vi "Periodic Tasks.vi"(8 "error in":errorcluster) -> ()   [LabVIEW 2016]
doc: "This VI runs in parallel to other tasks. It can contain as many user-defined periodic loops as you need. These can carry out PID or other sorts of timed response."
uses:
  <vilib>/addons/control/pid/pid.llb/PID Structure.ctl
  <vilib>/addons/control/pid/pid.llb/PID Time Unit.ctl
  <vilib>/addons/control/pid/pid.llb/PID Gain Unit.ctl
  Control 1.ctl
  <vilib>/Rock Robotics/WPI/ThirdParty/CanMotor/TalonSRX/WPI_CANTalonSRX_StatusFrame.ctl
  <vilib>/Rock Robotics/WPI/Solenoid/WPI_SolenoidValue.ctl
  <vilib>/Rock Robotics/WPI/Utilities/WPI_GetSetVariantRefNum.vi
  <vilib>/addons/control/pid/pid.llb/PID Structure Conversion (DBL).vi
  Robot Global Data.vi
  <vilib>/addons/control/pid/pid.llb/PID (DBL).vi
  <vilib>/addons/control/pid/pid.llb/PID Output Rate Limiter (DBL).vi
  <vilib>/Rock Robotics/WPI/RobotDrive/WPI_RobotDriveArcadeDrive_Standard(NoSaturation).vi
  <vilib>/Rock Robotics/Network Tables/NT Write Numeric Array.vi
  <vilib>/Rock Robotics/Network Tables/NT Write Number.vi
  <vilib>/Rock Robotics/Network Tables/NT Write Boolean.vi
  <vilib>/Rock Robotics/WPI/Solenoid/WPI_SolenoidSetEnum.vi
  <vilib>/Rock Robotics/WPI/Solenoid/Deprecated/WPI_SolenoidGetBool.vi
  <vilib>/addons/control/pid/NI_PID_pid.lvlib
panel:
  in  "BallIntakeCmd":dbl=0.45
  out "ANG-Input":dbl format="%#_3g"
  out "ANG-Output":dbl format="%#_3g"
  out "FWD-Output":dbl format="%#_3g"
  out "FWD-Input":dbl format="%#_3g"
  in  "ANG-A":dbl(slide)=0.7572815533980581 scale=0.0..1.0
  in  "ANG-B":dbl(slide)=0.3058252427184466 scale=0.0..1.0
  in  "FWD-B":dbl(slide)=0.24757281553398056 scale=0.0..1.0
  in  "FWD-A":dbl(slide)=0.12135922330097086 scale=0.0..1.0
  in  "DT Encoder Reset":bool
  in  "GearIntakeCmd":dbl=0.8
  in  "ShooterFlywCmd":dbl=8320.0
  in  "CtrlConv+UptReverse":bool
  in  "CtrlIntakeReverse":bool
  out "Flywheel Cmd & Speed":cluster{"Sensor Velocity":dbl}(graph)
  out "DTLeft - Under Voltage":bool
  out "DTLeft - Over Temp 2":bool
  out "DTRight- Over Temp":bool
  out "DTRight- Under Voltage":bool
  in  "output rate (EGU/min)":dbl=10000.0 format="%.2f"
  in  "P Fly":dbl=0.4
  in  "I Fly":dbl
  in  "D Fly":dbl
  in  "F Fly":dbl
  out "ShooterFlywThrottle":dbl
  out "ShooterFlywCur":dbl
  out "ShooterFlywEncVel":dbl
  out "ShooterFlywEncPos":dbl
  out "ShooterMasSensorVel":dbl
  out "ShooterFlywError":dbl
  in  "ShooterUptakeCmd":dbl=0.5
  out "ShooterUptakeSelection":bool
  out "ShooterUpCurr":dbl
  out "ShooterUpThrottle":dbl
  in  "ConveyorCmd":dbl=0.95
  out "DT Right Distance":dbl
  out "DT Encoder Avg":dbl
  out "Yaw Cmd & Angle":cluster{"Drive Angle":dbl, "Yaw":dbl}(graph)={"Drive Angle"=0.0, "Yaw"=-0.012991420041388195}
  out "PID gains F":T1
  out "PID gains A":T1
  out "DT Left/Right Motors":T2(graph)
  out "Arcade Y-Axis":dbl
  out "Arcade X-Axis":dbl
  out "Angle PID Out":dbl(graph)
  out "Fwd PID Out":dbl(graph)
  in  "Y-AxisJoyWgt":dbl=1.0
  in  "Fwd PID On":bool
  out "Fwd PIDoutput":dbl
  in  "PIDoutputRange F":cluster{"output high":dbl, "output low":dbl}={"output high"=0.8, "output low"=-0.8} {"output low" format="%.2f"; "output high" format="%.2f"}
  in  "ResetPID F":bool
  in  "derivative unit F":T3 items=["min", "s"]
  in  "proportional unit F":T4 items=["Gain (K)", "Band (PB)"]
  in  "integral unit F":T3 items=["min", "s"]
  in  "derivative F":dbl=4e-06
  in  "integral F":dbl=0.2
  in  "proportional F":dbl=0.002
  in  "Fwd PID structure":T5=1 items=["Academic (Standard)", "Parallel", "Series"]
  out "Angle PIDoutput":dbl
  in  "PIDoutputRange A":cluster{"output high":dbl, "output low":dbl}={"output high"=0.7, "output low"=-0.7} {"output low" format="%.2f"; "output high" format="%.2f"}
  in  "ResetAngle PID":bool
  in  "derivative unit A":T3 items=["min", "s"]
  in  "proportional unit A":T4 items=["Gain (K)", "Band (PB)"]
  in  "integral unit A":T3 items=["min", "s"]
  in  "derivative A":dbl=5e-05
  in  "integral A":dbl=11.0
  in  "proportional A":dbl=0.05
  in  "Angle PID structure":T5=1 items=["Academic (Standard)", "Parallel", "Series"]
  in  "DriveDistance Cmd":dbl
  out "DT Fwd Cmd & Right Encoder":cluster{"Drive Angle":dbl, "Yaw":dbl}(graph)={"Drive Angle"=0.0, "Yaw"=-0.012991420041388195}
  in  "Reset Gyro":bool
  out "Gyro Angle":dbl
  out "DT Left Distance":dbl
  out "DT Fwd Cmd & Left Encoder":cluster{"Drive Angle":dbl, "Yaw":dbl}(graph)={"Drive Angle"=0.0, "Yaw"=-0.012991420041388195}
  out "DT Encoder L-R":dbl(graph)
  out "DT Forward Cmd & Avg Distance":cluster{"Drive Angle":dbl, "Yaw":dbl}(graph)={"Drive Angle"=0.0, "Yaw"=-0.012991420041388195}
  out "Motor Values":dbl[](array[numeric])
  in  "X-AxisJoyWgt":dbl=0.8
  in  "Angle PID On":bool
  out "DTGearShiftHi":bool
  in  "DTClearStickyFaults":bool
  in  "DriveAngleCmd":dbl
  # "JOYSTICK SENSITIVITY COMPENSATION"
  # "P=0.025"
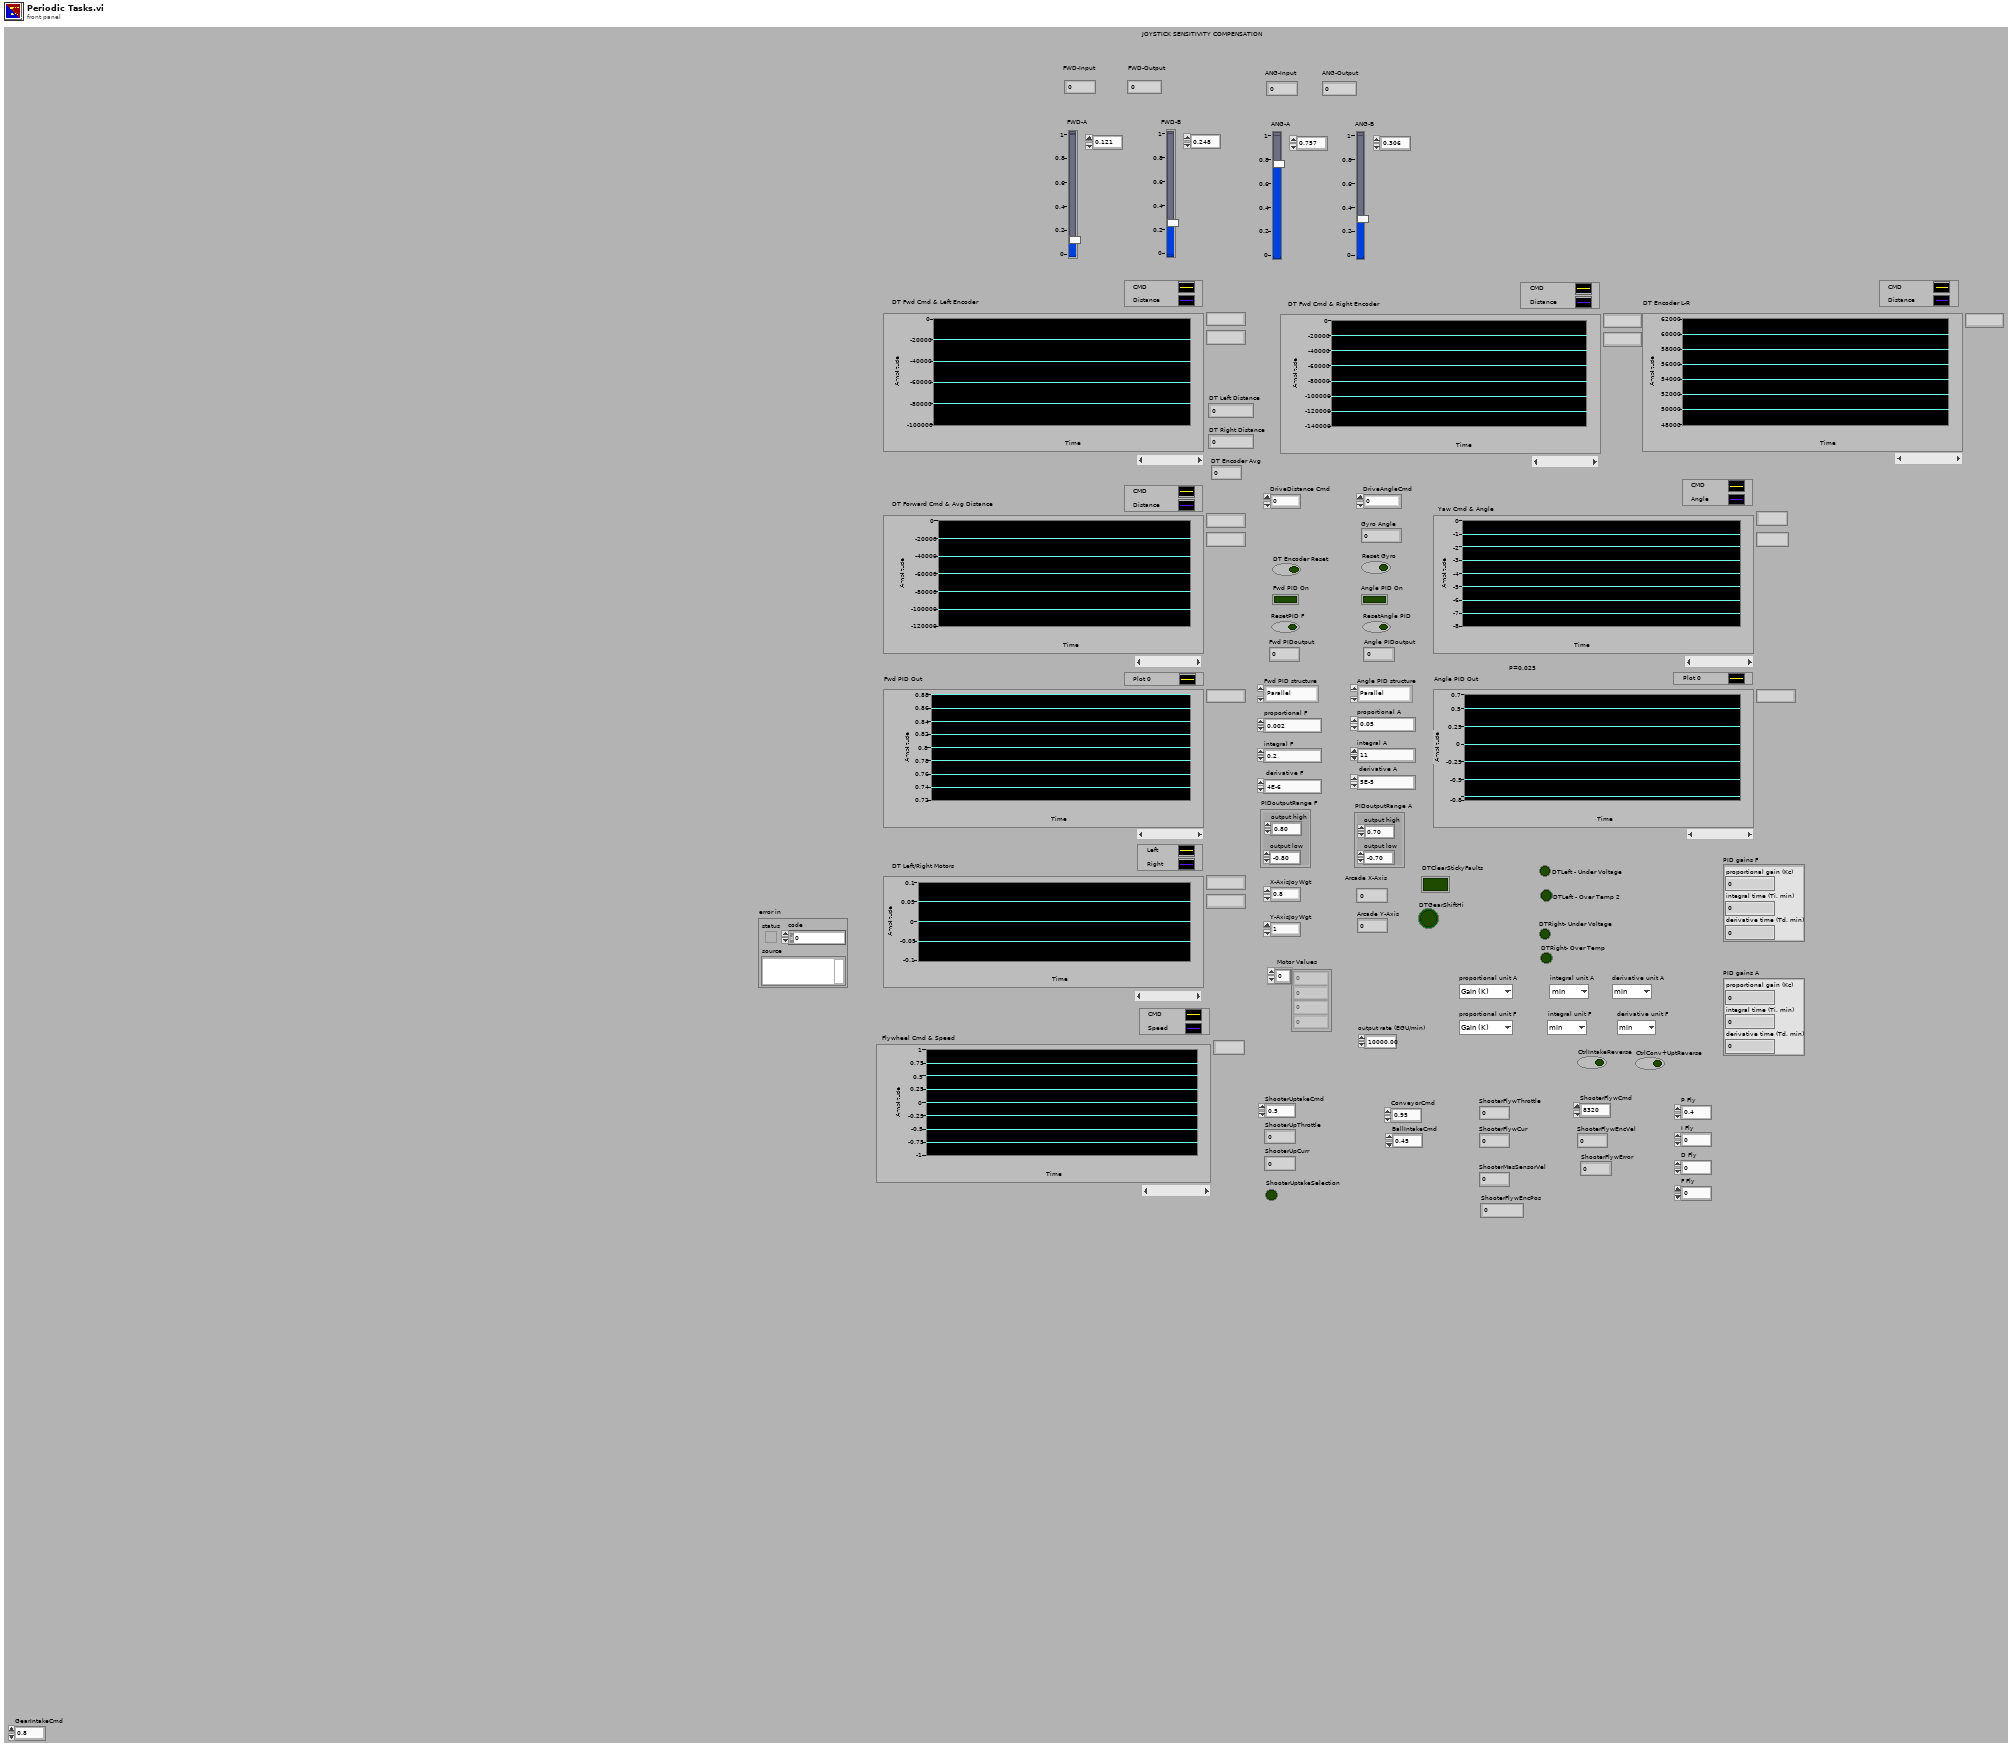
[diagram p1: front panel]
types:
  T1 = cluster{"proportional gain (Kc)":dbl, "integral time (Ti, min)":dbl, "derivative time (Td, min)":dbl}
  T2 = cluster{"Motor Values[0]":dbl, "Motor Values[1]":dbl}
  T3 = typedef "NI_PID_pid.lvlib/PID Time Unit.ctl" = u16
  T4 = typedef "NI_PID_pid.lvlib/PID Gain Unit.ctl" = u16
  T5 = typedef "NI_PID_pid.lvlib/PID Structure.ctl" = u16
  T6 = typedef "WPI_MotorControlDeviceRef.ctl" = cluster{"DeviceStatus":errorcluster, "Type":T7, "PWM":cluster{"PWM Channel":T8, "DeadBand":T9}, "CAN":cluster{"Device Number":u8, "SetOutput VI Ref":variant, "GetOutput VI Ref":variant, "Enable VI Ref":variant, "Disable VI Ref":variant, "Data":variant}, "Invert":bool}
  T7 = typedef "WPI_MotorControlType.ctl" = enum16{"PWM", "CAN"}
  T8 = typedef "FPGA_DIOPWMChannel.ctl" = enum8{"PWM 0", "PWM 1", "PWM 2", "PWM 3", "PWM 4", "PWM 5", "PWM 6", "PWM 7", "PWM 8", "PWM 9", "PWM MXP 0", "PWM MXP 1", "PWM MXP 2", "PWM MXP 3", "PWM MXP 4", "PWM MXP 5", "PWM MXP 6", "PWM MXP 7", "PWM MXP 8", "PWM MXP 9", "Invalid"}
  T9 = typedef "WPI_PWMDeadband.ctl" = cluster{"Name":string, "maxPositivePwm":i32, "minPositivePwm":i32, "centerPwm":i32, "maxNegativePwm":i32, "minNegativePwm":i32, "angularRange":u16}
  T10 = typedef "WPI_JoystickDevRef.ctl" = cluster{"Device":T11}
  T11 = typedef "WPI_JoystickDeviceEnum.ctl" = enum16{"USB 0", "USB 1", "USB 2", "USB 3", "USB 4", "USB 5"}
  T12 = typedef "WPI_RobotDriveDevRef.ctl" = cluster{"DevStatus":errorcluster, "Motors[]":T6[], "Square Inputs":bool, "Max Output":dbl}
  T13 = cluster{"MotorControlDevRef":T6, "JoystickDevRef":T10, "RobotDriveDevRef":T12}
  T14 = typedef "WPI_SolenoidDevRef.ctl" = cluster{"DevStatus":errorcluster, "Pneumatics Control Module":u8, "Forward Solenoid Channel":T15, "Reverse Solenoid Channel":T15}
  T15 = typedef "WPI_SolenoidChannel.ctl" = enum8{"Solenoid 0", "Solenoid 1", "Solenoid 2", "Solenoid 3", "Solenoid 4", "Solenoid 5", "Solenoid 6", "Solenoid 7", "Invalid"}
  T16 = typedef "WPI_GyroDevRef.ctl" = cluster{"DevStatus":errorcluster, "Analog Channel":T17, "Offset":dbl, "Gain (VoltsPerDegree/Second)":dbl, "Gyro Type":enum16{"Analog", "XRS450"}, "Handle":i32, "SPI Bus":T18, "Device Found":bool, "Sample Rate":dbl, "Calibrate On Open":bool}
  T17 = typedef "FPGA_AIChannel.ctl" = enum8{"AI 0", "AI 1", "AI 2", "AI 3", "AI MXP 0", "AI MXP 1", "AI MXP 2", "AI MXP 3", "Invalid"}
  T18 = typedef "spi_bus.ctl" = enum16{"SPI On-Board, CS0", "SPI On-Board, CS1", "SPI On-Board, CS2", "SPI On-Board, CS3", "SPI MXP", "Invalid"}
  T19 = typedef "WPI_SolenoidValue.ctl" = enum16{"Off", "On", "Forward", "Reverse"}
  T20 = typedef "WPI_CANTalonSRX_GlobalStatus.ctl" = cluster{"Applied Throttle":dbl, "Module Enabled":bool, "CAN Error":errorcluster, "Closed Loop Error":dbl, "Forward Limit Switch Closed":bool, "Reverse Limit Switch Closed":bool, "Sensor Position":dbl, "Sensor Velocity":dbl, "Current":dbl, "Sticky Fault - Over Temp":bool, "Sticky Fault - Under Voltage":bool, "Sticky Fault - Forward Limit":bool, "Sticky Fault - Reverse Limit":bool, "Sticky Fault - Forward Soft Limit":bool, "Sticky Fault - Reverse Soft Limit":bool, "Brake is Enabled":bool, "Encoder Position":dbl, "Encoder Velocity":dbl, "Encoder Index Count":dbl, "Encoder A Pin State":bool, "Encoder B Pin State":bool, "Encoder Index Pin State":bool, "Analog In":dbl, "Analog In Velocity":dbl, "Temperature (C)":dbl, "Battery Voltage":dbl, "Control 5 Is Supported":bool, "Current Profile Slot Select":dbl, "Pos Div 8":bool, "Vel Div 4":bool, "Pulse Width Position":i32, "Pulse Width Velocity":i32, "Pulse Width Rise To Rise (us)":i32, "Pulse Width Rise To Fall (us)":i32, "Mot Prof Active Is Under Run":bool, "Mot Prof Active Has Under Run":bool, "Mot Prof Active Is Last":bool, "Mot Prof Active Velocity Only":bool, "Mot Prof Active Is Valid":bool, "Mot Prof Buffer Is Full":bool, "Mot Prof Active Profile Slot Select":i32, "Mot Prof NextID":i32, "Mot Prof Count":i32, "Mot Prof Active Velocity":dbl, "Mot Prof Active Position":dbl, "Mot Prof Output Enable":i32}
  T21 = cluster{"Motor Values[0]":dbl, "Motor Values[1]":dbl, "Motor Values[2]":dbl, "Motor Values[3]":dbl, "Motor Values[4]":dbl, "Motor Values[5]":dbl, "Motor Values[6]":dbl, "Motor Values[7]":dbl, "Motor Values[8]":dbl}
  T22 = enum16{"Start", "Search", "Secure", "Release", "Standby", "Wait", "Wait Release"}
  T23 = typedef "Control 1.ctl" = enum16{"Autonomous Disabled", "Autonomous Enabled", "Teleop Disabled", "Teleop Enabled", "Disconnected", "Finish", "Test Disabled", "Test Enabled", "Emergency Stopped"}
  T24 = cluster{"Buttons[0]":bool, "Buttons[1]":bool, "Buttons[2]":bool, "Buttons[3]":bool, "Buttons[4]":bool, "Buttons[5]":bool, "Buttons[6]":bool, "Buttons[7]":bool, "Buttons[8]":bool}
  T25 = cluster{"Axes[0]":dbl, "Axes[1]":dbl, "Axes[2]":dbl, "Axes[3]":dbl, "Axes[4]":dbl, "Axes[5]":dbl, "Axes[6]":dbl, "Axes[7]":dbl, "Axes[8]":dbl}
  T26 = typedef "WPI_DriverStationRobotMode2.ctl" = enum16{"Autonomous Disabled", "Autonomous Enabled", "Teleop Disabled", "Teleop Enabled", "Disconnected", "Finish", "Test Disabled", "Test Enabled", "Emergency Stopped"}
  T27 = typedef "WPI_CANTalonSRX_StatusFrame.ctl" = enum16{"General Status Frame", "Feedback Status Frame", "Quadrature Status Frame", "Analog Temp Vbat Status Frame", "Pulse Width Status Frame"}
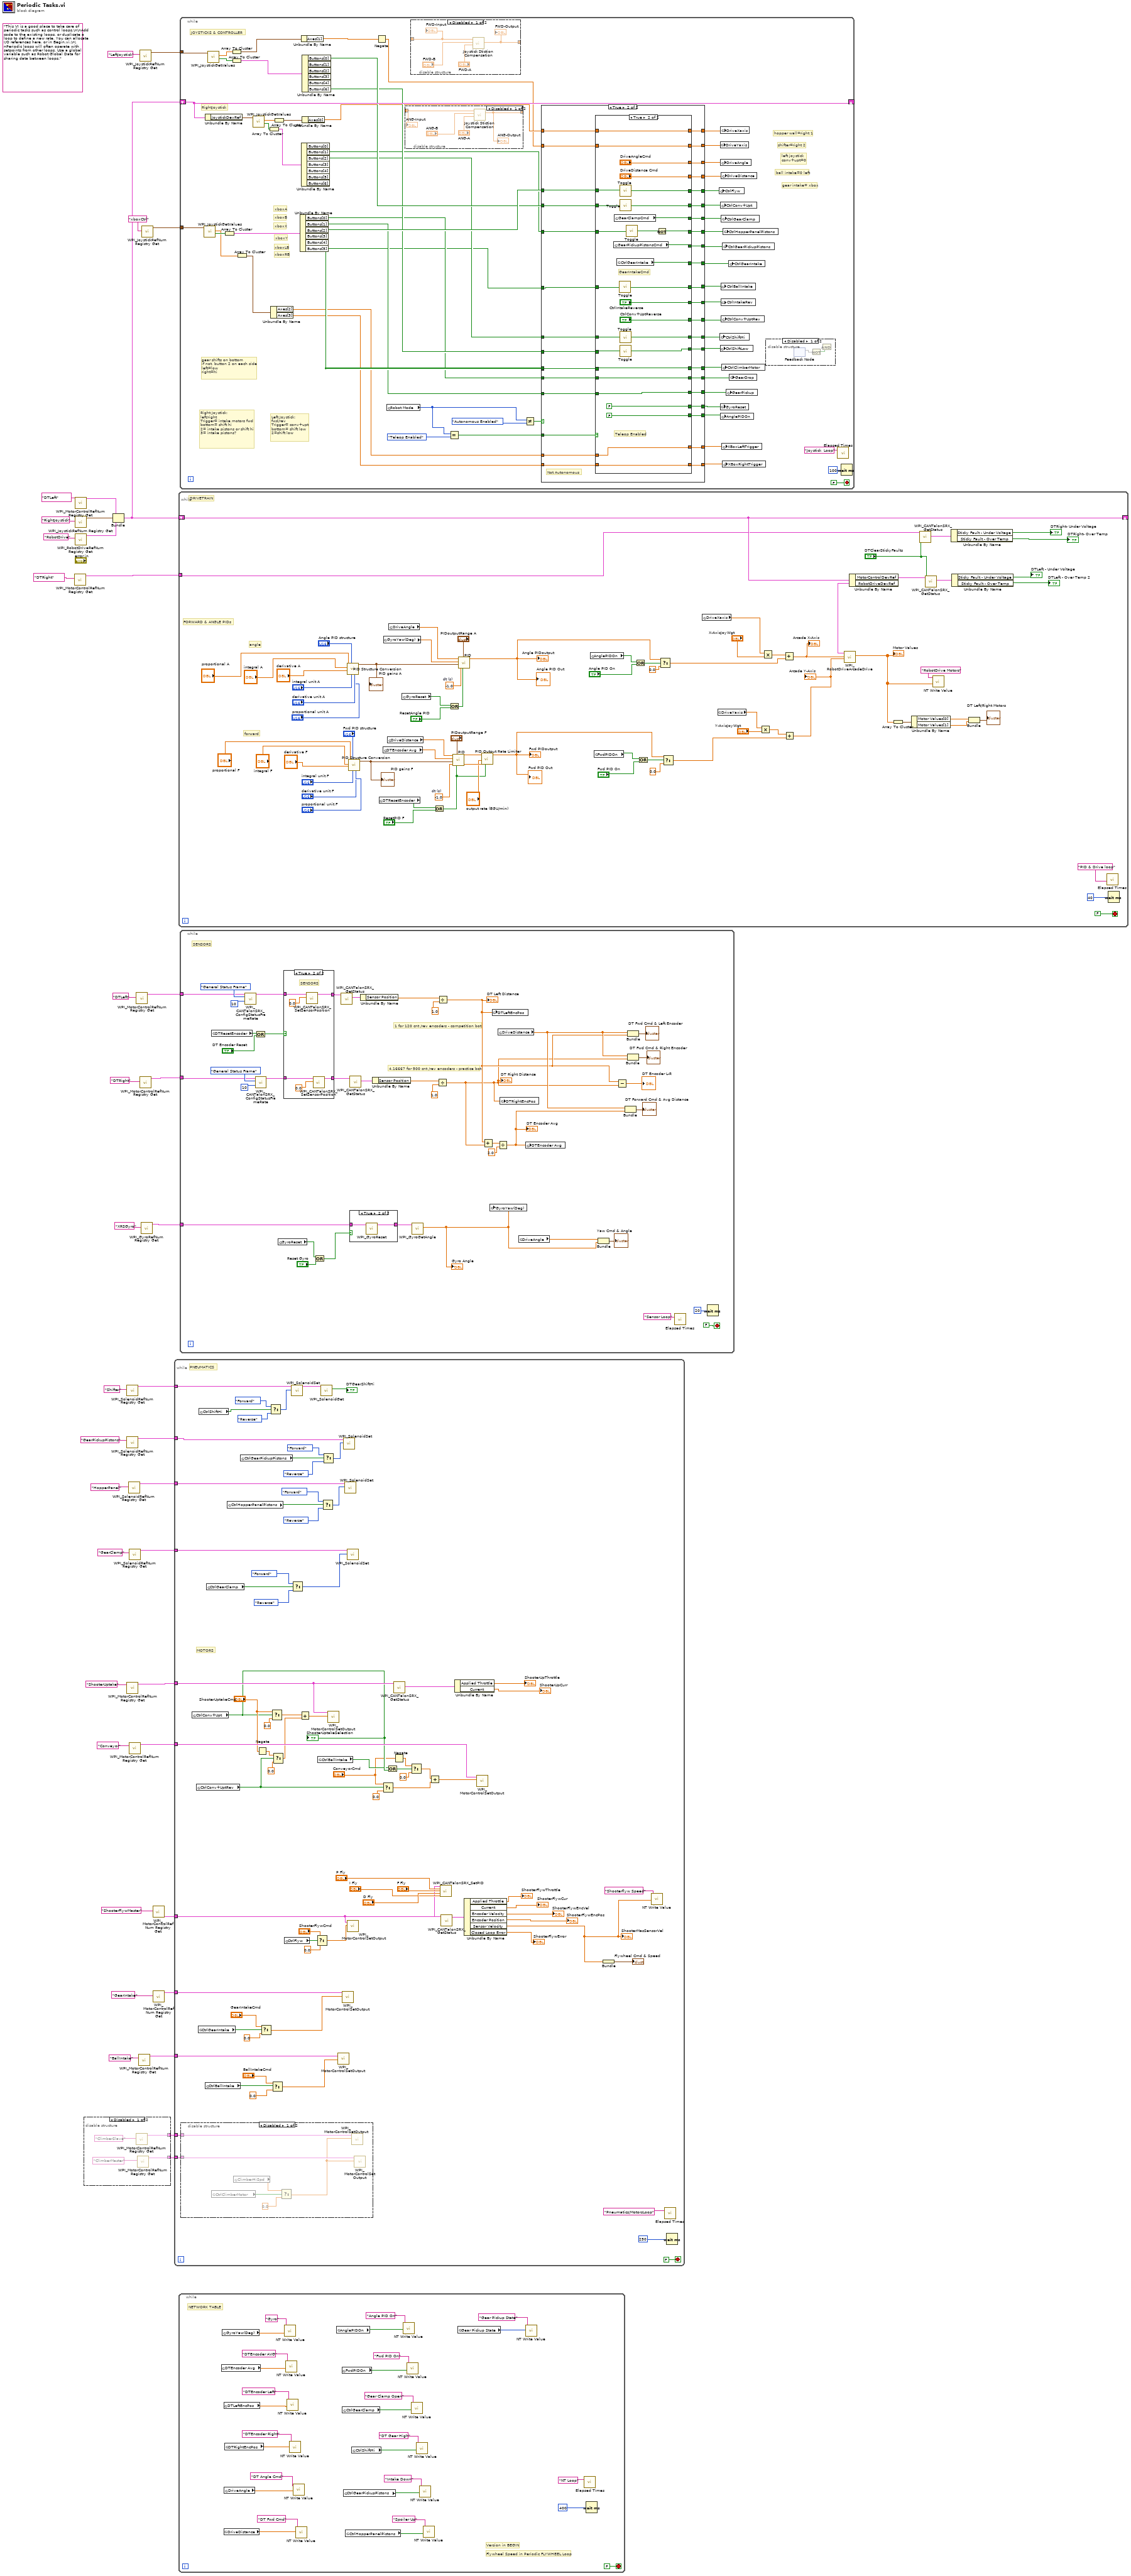
[diagram p0: block diagram]
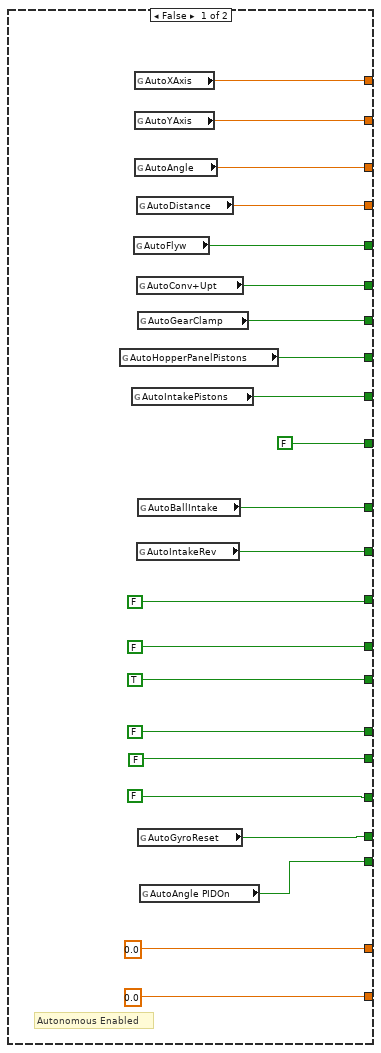
[diagram p9: hidden frame]
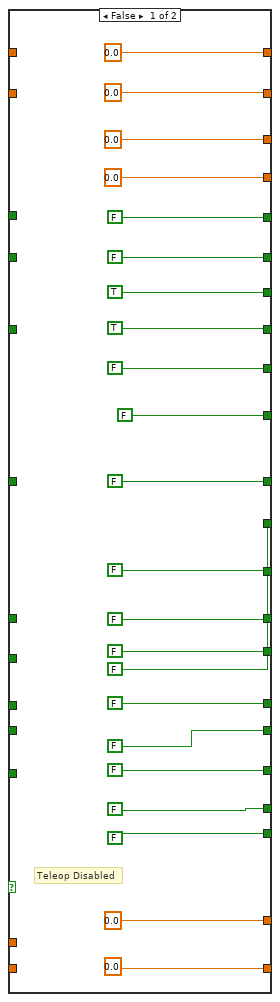
[diagram p10: hidden frame]
diagram:
  (unwired) "This VI is a good place to take care of periodic tasks such as control loops.\n\nAdd code to the existing loops, or duplicate a loop to define a new rate. You can allocate I/O references here, or in Begin.vi.\n\nPeriodic loops will often operate with setpoints from other loops. Use a global variable such as Robot Global Data for sharing data between loops."
  n1 = call <vilib>:"WPI_MotorControlRefNum Registry Get.vi"("refnum name"="DTRight") -> ("MotorControlDevRef"=w28:T6)  [unwired: 9 in, 1 out]
  n2 = call <vilib>:"WPI_MotorControlRefNum Registry Get.vi"("refnum name"="DTLeft") -> ("MotorControlDevRef"=w30:T6)  [unwired: 9 in, 1 out]
  n3 = call <vilib>:"WPI_JoystickRefNum Registry Get.vi"("refnum name"="RightJoystick") -> ("JoystickDevRef"=w37:T10)  [unwired: 1 in, 9 out]
  n4 = call <vilib>:"WPI_RobotDriveRefNum Registry Get.vi"("refnum name"="RobotDrive") -> ("RobotDriveDevRef"=w36:T12)  [unwired: 1 in, 9 out]
  n5 = disable-structure shown="Disabled" {
    disable-tunnel: [w41 _] -> w4
    disable-tunnel: [w40 _] -> w3
    frame Disabled {
      n6 = call <vilib>:"WPI_MotorControlRefNum Registry Get.vi"("refnum name"="ClimberSlave") -> ("MotorControlDevRef"=w41:T6)  [unwired: 9 in, 1 out]
      n7 = call <vilib>:"WPI_MotorControlRefNum Registry Get.vi"("refnum name"="ClimberMaster") -> ("MotorControlDevRef"=w40:T6)  [unwired: 9 in, 1 out]
    }
    frame Enabled {
    }
  }
  n8 = Bundle("MotorControlDevRef"=w30, "JoystickDevRef"=w37, "RobotDriveDevRef"=w36) -> (w35:T13)  [unwired: 1 out]
  n9 = call <vilib>:"WPI_SolenoidRefNum Registry Get.vi"("refnum name"="Shifter") -> ("SolenoidDevRef"=w25:T14)  [unwired: 9 in, 1 out]
  n10 = call <vilib>:"WPI_SolenoidRefNum Registry Get.vi"("refnum name"="GearPickupPistons") -> ("SolenoidDevRef"=w17:T14)  [unwired: 9 in, 1 out]
  n11 = call <vilib>:"WPI_MotorControlRefNum Registry Get.vi"("refnum name"="ShooterUptake") -> ("MotorControlDevRef"=w20:T6)  [unwired: 9 in, 1 out]
  n12 = call <vilib>:"WPI_SolenoidRefNum Registry Get.vi"("refnum name"="HopperPanel") -> ("SolenoidDevRef"=w23:T14)  [unwired: 9 in, 1 out]
  n13 = call <vilib>:"WPI_SolenoidRefNum Registry Get.vi"("refnum name"="GearClamp") -> ("SolenoidDevRef"=w15:T14)  [unwired: 9 in, 1 out]
  n14 = call <vilib>:"WPI_MotorControlRefNum Registry Get.vi"("refnum name"="Conveyor") -> ("MotorControlDevRef"=w19:T6)  [unwired: 9 in, 1 out]
  n15 = call <vilib>:"WPI_MotorControlRefNum Registry Get.vi"("refnum name"="DTLeft") -> ("MotorControlDevRef"=w9:T6)  [unwired: 9 in, 1 out]
  n16 = call <vilib>:"WPI_MotorControlRefNum Registry Get.vi"("refnum name"="BallIntake") -> ("MotorControlDevRef"=w1:T6)  [unwired: 9 in, 1 out]
  n17 = call <vilib>:"WPI_JoystickRefNum Registry Get.vi"("refnum name"="LeftJoystick") -> ("JoystickDevRef"=w33:T10)  [unwired: 1 in, 9 out]
  n18 = call <vilib>:"WPI_MotorControlRefNum Registry Get.vi"("refnum name"="DTRight") -> ("MotorControlDevRef"=w8:T6)  [unwired: 9 in, 1 out]
  n19 = call <vilib>:"WPI_GyroRefNum Registry Get.vi"("refnum name"="XRSGyro") -> ("GyroDevRef"=w11:T16)  [unwired: 9 in, 1 out]
  n20 = call <vilib>:"WPI_JoystickRefNum Registry Get.vi"("refnum name"="xboxCtrl") -> ("JoystickDevRef"=w26:T10)  [unwired: 1 in, 9 out]
  n21 = call <vilib>:"WPI_MotorControlRefNum Registry Get.vi"("refnum name"="ShooterFlywMaster") -> ("MotorControlDevRef"=w13:T6)  [unwired: 9 in, 1 out]
  n22 = call <vilib>:"WPI_MotorControlRefNum Registry Get.vi"("refnum name"="GearIntake") -> ("MotorControlDevRef"=w5:T6)  [unwired: 9 in, 1 out]
  n23 = while {
    tunnel: w25 -> [w122]
    tunnel: w23 -> [w121]
    tunnel: w20 -> [w120]
    tunnel: w19 -> [w119]
    tunnel: w17 -> [w118]
    tunnel: w15 -> [w117]
    tunnel: w13 -> [w116]
    tunnel: w5 -> [w115]
    tunnel: w4 -> [w114]
    tunnel: w3 -> [w113]
    tunnel: w1 -> [w112]
    stop <- FALSE stop-if-true
    # "PNEUMATICS"
    # "MOTORS"
    n24 = disable-structure shown="Disabled" {
      disable-tunnel: w114 -> [w128 _]
      disable-tunnel: w113 -> [w127 _]
      frame Disabled {
        n25 = global read "Robot Global Data.vi" "CtrlClimberMotor"() -> (w124:bool)
        n26 = global read "Robot Global Data.vi" "ClimberHiSpd"() -> (w125:dbl)
        n27 = Select(t=w125, s=w124, f=0.0) -> (s? t:f=w123:dbl)
        n28 = call <vilib>:"WPI_MotorControlSetOutput.vi"("Output"=w123, "MotorControlDevRef"=w128) -> ()  [unwired: 7 in, 3 out]
        n29 = call <vilib>:"WPI_MotorControlSetOutput.vi"("Output"=w123, "MotorControlDevRef"=w127) -> ()  [unwired: 7 in, 3 out]
      }
      frame Enabled {
      }
    }
    n30 = global read "Robot Global Data.vi" "CtrlConv+Upt"() -> (w94:bool)
    "ShooterUptakeSelection" <- w94
    n31 = global read "Robot Global Data.vi" "CtrlConv+UptRev"() -> (w111:bool)
    n32 = global read "Robot Global Data.vi" "CtrlGearIntake"() -> (w52:bool)
    n33 = global read "Robot Global Data.vi" "CtrlShiftHi"() -> (w78:bool)
    n34 = global read "Robot Global Data.vi" "CtrlBallIntake"() -> (w47:bool)
    n35 = global read "Robot Global Data.vi" "CtrlGearClamp"() -> (w77:bool)
    n36 = global read "Robot Global Data.vi" "CtrlHopperPanelPistons"() -> (w79:bool)
    n37 = global read "Robot Global Data.vi" "CtrlGearPickupPistons"() -> (w80:bool)
    n38 = Negate(x="ShooterUptakeCmd") -> (-x=w108:dbl)
    n39 = Select(t="GearIntakeCmd", s=w52, f=0.0) -> (s? t:f=w54:dbl)
    n40 = Select(t=WPI_SolenoidValue."Forward" ("Value"), s=w78, f=WPI_SolenoidValue."Reverse" ("Value")) -> (s? t:f=w88:T19)
    n41 = Select(t="ShooterUptakeCmd", s=w94, f=0.0) -> (s? t:f=w104:dbl)
    n42 = Select(t="BallIntakeCmd", s=w47, f=0.0) -> (s? t:f=w50:dbl)
    n43 = Select(t=w108, s=w111, f=0.0) -> (s? t:f=w105:dbl)
    n44 = global read "Robot Global Data.vi" "CtrlFlyw"() -> (w58:bool)
    n45 = call-poly <vilib>:"WPI_SolenoidSet.vi"("Value"=w88, "SolenoidDevRef"=w122) -> ("SolenoidDevRef"=w87:T14)  [unwired: 8 in, 1 out]
    n46 = Select(t=WPI_SolenoidValue."Forward" ("Value"), s=w77, f=WPI_SolenoidValue."Reverse" ("Value")) -> (s? t:f=w74:T19)
    n47 = Add(x=w104, y=w105) -> (x+y=w109:dbl)
    n48 = Select(t="ShooterFlywCmd", s=w58, f=0.0) -> (s? t:f=w55:dbl)
    n49 = global read "Robot Global Data.vi" "CtrlBallIntake"() -> (w93:bool)
    n50 = call-poly <vilib>:"WPI_SolenoidGet.vi"("SolenoidDevRef"=w87) -> ("Value"=→"DTGearShiftHi":bool)  [unwired: 8 in, 2 out]
    n51 = Select(t=WPI_SolenoidValue."Forward" ("Value"), s=w79, f=WPI_SolenoidValue."Reverse" ("Value")) -> (s? t:f=w83:T19)
    n52 = Select(t=WPI_SolenoidValue."Forward" ("Value"), s=w80, f=WPI_SolenoidValue."Reverse" ("Value")) -> (s? t:f=w82:T19)
    n53 = call <vilib>:"WPI_MotorControlSetOutput.vi"("Output"=w109, "MotorControlDevRef"=w120) -> ()  [unwired: 7 in, 3 out]
    n54 = call <vilib>:"WPI_MotorControlSetOutput.vi"("Output"=w50, "MotorControlDevRef"=w112) -> ()  [unwired: 7 in, 3 out]
    n55 = call <vilib>:"WPI_MotorControlSetOutput.vi"("Output"=w54, "MotorControlDevRef"=w115) -> ()  [unwired: 7 in, 3 out]
    n56 = call-poly <vilib>:"WPI_SolenoidSet.vi"("Value"=w82, "SolenoidDevRef"=w118) -> ()  [unwired: 8 in, 2 out]
    n57 = call-poly <vilib>:"WPI_SolenoidSet.vi"("Value"=w83, "SolenoidDevRef"=w121) -> ()  [unwired: 8 in, 2 out]
    n58 = call-poly <vilib>:"WPI_SolenoidSet.vi"("Value"=w74, "SolenoidDevRef"=w117) -> ()  [unwired: 8 in, 2 out]
    n59 = call <vilib>:"WPI_MotorControlSetOutput.vi"("Output"=w55, "MotorControlDevRef"=w116) -> ()  [unwired: 7 in, 3 out]
    n60 = Select(t="ConveyorCmd", s=w111, f=0.0) -> (s? t:f=w97:dbl)
    n61 = Or(x=w93, y=w94) -> (x .or. y?=w92:bool)
    n62 = Negate(x="ConveyorCmd") -> (-x=w98:dbl)
    n63 = call <vilib>:"WPI_CANTalonSRX_GetStatus.vi"("CAN Talon SRX Ref"=w120) -> ("Talon SRX Status"=w100:T20)  [unwired: 8 in, 2 out]
    n64 = Select(t=w98, s=w92, f=0.0) -> (s? t:f=w101:dbl)
    n65 = Add(x=w101, y=w97) -> (x+y=w103:dbl)
    n66 = call <vilib>:"WPI_CANTalonSRX_GetStatus.vi"("CAN Talon SRX Ref"=w116) -> ("Talon SRX Status"=w67:T20, "CAN Talon SRX Ref"=w62:T6)  [unwired: 8 in, 1 out]
    n67 = call <vilib>:"WPI_CANTalonSRX_SetPID.vi"("CAN Talon SRX Ref"=w62, "P"="P Fly", "I"="I Fly", "D"="D Fly", "F"="F Fly") -> ()  [unwired: 9 in, 2 out]
    n68 = Unbundle By Name(w100) -> ("Applied Throttle"=→"ShooterUpThrottle":dbl, "Current"=→"ShooterUpCurr":dbl)
    n69 = Unbundle By Name(w67) -> ("Applied Throttle"=→"ShooterFlywThrottle":dbl, "Current"=→"ShooterFlywCur":dbl, "Encoder Velocity"=→"ShooterFlywEncVel":dbl, "Encoder Position"=→"ShooterFlywEncPos":dbl, "Sensor Velocity"=w59:dbl, "Closed Loop Error"=→"ShooterFlywError":dbl)
    "ShooterMasSensorVel" <- w59
    n70 = call <vilib>:"WPI_MotorControlSetOutput.vi"("Output"=w103, "MotorControlDevRef"=w119) -> ()  [unwired: 7 in, 3 out]
    n71 = Bundle("Sensor Velocity"=w59) -> (→"Flywheel Cmd & Speed":cluster{"Sensor Velocity":dbl})  [unwired: 1 in]
    n72 = call-poly <vilib>:"NT Write Value.vi"("Numeric"=w59, "Name"="Shooterflyw Speed") -> ()  [unwired: 9 in, 1 out]
    n73 = call "Elapsed Times.vi"("Call Name"="Pneumatics/MotorsLoop") -> ()  [unwired: 2 in, 1 out]
    n74 = Wait (ms)(milliseconds to wait=u32 250) -> ()  [unwired: 1 out]
  }
  n75 = while {
    shift-right: [w200] -> _
    shift-left: w35 -> [w200]
    tunnel: w28 -> [w191]
    stop <- FALSE stop-if-true
    w152 = -1.0  # dt (s)
    w137 = -1.0  # dt (s)
    # "FORWARD & ANGLE PIDs"
    # "angle"
    # "forward"
    # "DRIVETRAIN"
    n76 = call-poly <vilib>:"PID Structure Conversion.vi"("derivative unit"="derivative unit A", "proportional unit"="proportional unit A", "integral unit"="integral unit A", "PID structure"="Angle PID structure", "derivative"="derivative A", "integral"="integral A", "proportional"="proportional A") -> ("PID gains"=w150:T1)  [unwired: 4 in]
    "PID gains A" <- w150
    n77 = call-poly <vilib>:"PID Structure Conversion.vi"("derivative unit"="derivative unit F", "proportional unit"="proportional unit F", "integral unit"="integral unit F", "PID structure"="Fwd PID structure", "derivative"="derivative F", "integral"="integral F", "proportional"="proportional F") -> ("PID gains"=w133:T1)  [unwired: 4 in]
    "PID gains F" <- w133
    n78 = global read "Robot Global Data.vi" "DTResetEncoder"() -> (w138:bool)
    n79 = global read "Robot Global Data.vi" "DTEncoder Avg"() -> (w134:dbl)
    n80 = global read "Robot Global Data.vi" "GyroYaw(Deg)"() -> (w151:dbl)
    n81 = global read "Robot Global Data.vi" "DriveDistance"() -> (w136:dbl)
    n82 = global read "Robot Global Data.vi" "DriveAngle"() -> (w147:dbl)
    n83 = global read "Robot Global Data.vi" "GyroReset"() -> (w154:bool)
    n84 = Or(x=w138, y="ResetPID F") -> (x .or. y?=w129:bool)
    n85 = Or(x=w154, y="ResetAngle PID") -> (x .or. y?=w153:bool)
    n86 = call-poly <vilib>:"PID.vi"("reinitialize? (F)"=w129, "output range"="PIDoutputRange F", "dt (s)"=w137, "PID gains"=w133, "process variable"=w134, "setpoint"=w136) -> ("dt out (s)"=w131:dbl, "output"=w132:dbl)  [unwired: 4 in]
    n87 = call-poly <vilib>:"PID.vi"("reinitialize? (F)"=w153, "output range"="PIDoutputRange A", "dt (s)"=w152, "PID gains"=w150, "process variable"=w151, "setpoint"=w147) -> ("output"=w163:dbl)  [unwired: 4 in, 1 out]
    "Angle PIDoutput" <- w163
    "Angle PID Out" <- w163
    n88 = call-poly <vilib>:"PID Output Rate Limiter.vi"("reinitialize? (F)"=w129, "dt (s)"=w131, "output rate (EGU/min)"="output rate (EGU/min)", "input (controller output)"=w132) -> ("output"=w162:dbl)  [unwired: 4 in, 1 out]
    "Fwd PIDoutput" <- w162
    "Fwd PID Out" <- w162
    n89 = global read "Robot Global Data.vi" "AnglePIDOn"() -> (w171:bool)
    n90 = global read "Robot Global Data.vi" "FwdPIDOn"() -> (w165:bool)
    n91 = Or(x=w171, y="Angle PID On") -> (x .or. y?=w169:bool)
    n92 = Or(x=w165, y="Fwd PID On") -> (x .or. y?=w167:bool)
    n93 = Select(t=w163, s=w169, f=0.0) -> (s? t:f=w177:dbl)
    n94 = Select(t=w162, s=w167, f=0.0) -> (s? t:f=w189:dbl)
    n95 = global read "Robot Global Data.vi" "DriveXaxis"() -> (w198:dbl)
    n96 = global read "Robot Global Data.vi" "DriveYaxis"() -> (w186:dbl)
    n97 = Multiply(x=w186, y="Y-AxisJoyWgt") -> (x*y=w188:dbl)
    n98 = Multiply(x=w198, y="X-AxisJoyWgt") -> (x*y=w196:dbl)
    n99 = Add(x=w196, y=w177) -> (x+y=w184:dbl)
    "Arcade X-Axis" <- w184
    n100 = Add(x=w188, y=w189) -> (x+y=w185:dbl)
    "Arcade Y-Axis" <- w185
    n101 = Unbundle By Name(w200) -> ("MotorControlDevRef"=w192:T6, "RobotDriveDevRef"=w194:T12)
    n102 = call-poly <vilib>:"WPI_RobotDriveArcadeDrive.vi"("Y axis value"=w185, "X axis value"=w184, "RobotDriveDevRef"=w194) -> ("Motor Values"=w183:dbl[])  [unwired: 6 in, 2 out]
    "Motor Values" <- w183
    n103 = Array To Cluster(array=w183) -> (cluster=w182:T21)
    n104 = Unbundle By Name(w182) -> ("Motor Values[0]"=w181:dbl, "Motor Values[1]"=w180:dbl)
    n105 = call <vilib>:"WPI_CANTalonSRX_GetStatus.vi"("Clear Sticky Faults"="DTClearStickyFaults", "CAN Talon SRX Ref"=w191) -> ("Talon SRX Status"=w195:T20)  [unwired: 7 in, 2 out]
    n106 = call <vilib>:"WPI_CANTalonSRX_GetStatus.vi"("Clear Sticky Faults"="DTClearStickyFaults", "CAN Talon SRX Ref"=w192) -> ("Talon SRX Status"=w193:T20)  [unwired: 7 in, 2 out]
    n107 = call-poly <vilib>:"NT Write Value.vi"("Numeric Array"=w183, "Name"="RobotDrive Motors") -> ()  [unwired: 9 in, 1 out]
    n108 = Unbundle By Name(w195) -> ("Sticky Fault - Under Voltage"=→"DTRight- Under Voltage":bool, "Sticky Fault - Over Temp"=→"DTRight- Over Temp":bool)
    n109 = Unbundle By Name(w193) -> ("Sticky Fault - Under Voltage"=→"DTLeft - Under Voltage":bool, "Sticky Fault - Over Temp"=→"DTLeft - Over Temp 2":bool)
    n110 = Bundle("Motor Values[0]"=w181, "Motor Values[1]"=w180) -> (→"DT Left/Right Motors":T2)  [unwired: 1 in]
    n111 = call "Elapsed Times.vi"("Call Name"="PID & Drive loop") -> ()  [unwired: 2 in, 1 out]
    n112 = Wait (ms)(milliseconds to wait=u32 40) -> ()  [unwired: 1 out]
  }
  n113 = while {
    stop <- FALSE stop-if-true
    # "NETWORK TABLE"
    # "Version in BEGIN"
    # "Flywheel Speed in Periodic FLYWHEEL Loop"
    n114 = global read "Robot Global Data.vi" "DTEncoder Avg"() -> (w226:dbl)
    n115 = global read "Robot Global Data.vi" "GyroYaw(Deg)"() -> (w225:dbl)
    n116 = global read "Robot Global Data.vi" "DTLeftEncPos"() -> (w227:dbl)
    n117 = global read "Robot Global Data.vi" "DriveDistance"() -> (w230:dbl)
    n118 = global read "Robot Global Data.vi" "DriveAngle"() -> (w229:dbl)
    n119 = global read "Robot Global Data.vi" "DTRightEncPos"() -> (w228:dbl)
    n120 = call-poly <vilib>:"NT Write Value.vi"("Numeric"=w225, "Name"="Gyro") -> ()  [unwired: 9 in, 1 out]
    n121 = call-poly <vilib>:"NT Write Value.vi"("Numeric"=w226, "Name"="DTEncoder AVG") -> ()  [unwired: 9 in, 1 out]
    n122 = call-poly <vilib>:"NT Write Value.vi"("Numeric"=w227, "Name"="DTEncoder Left") -> ()  [unwired: 9 in, 1 out]
    n123 = call-poly <vilib>:"NT Write Value.vi"("Numeric"=w228, "Name"="DTEncoder Right") -> ()  [unwired: 9 in, 1 out]
    n124 = call-poly <vilib>:"NT Write Value.vi"("Numeric"=w229, "Name"="DT Angle Cmd") -> ()  [unwired: 9 in, 1 out]
    n125 = call-poly <vilib>:"NT Write Value.vi"("Numeric"=w230, "Name"="DT Fwd Cmd") -> ()  [unwired: 9 in, 1 out]
    n126 = global read "Robot Global Data.vi" "AnglePIDOn"() -> (w208:bool)
    n127 = global read "Robot Global Data.vi" "FwdPIDOn"() -> (w209:bool)
    n128 = global read "Robot Global Data.vi" "CtrlGearClamp"() -> (w218:bool)
    n129 = global read "Robot Global Data.vi" "CtrlGearPickupPistons"() -> (w214:bool)
    n130 = global read "Robot Global Data.vi" "CtrlHopperPanelPistons"() -> (w215:bool)
    n131 = global read "Robot Global Data.vi" "CtrlShiftHi"() -> (w212:bool)
    n132 = call-poly <vilib>:"NT Write Value.vi"("Boolean"=w208, "Name"="Angle PID On") -> ()  [unwired: 9 in, 1 out]
    n133 = call-poly <vilib>:"NT Write Value.vi"("Boolean"=w209, "Name"="Fwd PID On") -> ()  [unwired: 9 in, 1 out]
    n134 = call-poly <vilib>:"NT Write Value.vi"("Boolean"=w218, "Name"="Gear Clamp Open") -> ()  [unwired: 9 in, 1 out]
    n135 = call-poly <vilib>:"NT Write Value.vi"("Boolean"=w212, "Name"="DT Gear High") -> ()  [unwired: 9 in, 1 out]
    n136 = call-poly <vilib>:"NT Write Value.vi"("Boolean"=w214, "Name"="Intake Down") -> ()  [unwired: 9 in, 1 out]
    n137 = call-poly <vilib>:"NT Write Value.vi"("Boolean"=w215, "Name"="Spoiler Up") -> ()  [unwired: 9 in, 1 out]
    n138 = global read "Robot Global Data.vi" "Gear Pickup State"() -> (w205:T22)
    n139 = call-poly <vilib>:"NT Write Value.vi"("Numeric"=w205, "Name"="Gear Pickup State") -> ()  [unwired: 9 in, 1 out]
    n140 = call "Elapsed Times.vi"("Call Name"="NT Loop") -> ()  [unwired: 2 in, 1 out]
    n141 = Wait (ms)(milliseconds to wait=u32 400) -> ()  [unwired: 1 out]
  }
  n142 = while {
    shift-right: [w288] -> _
    shift-left: w35 -> [w288]
    tunnel: w33 -> [w285]
    tunnel: w26 -> [w272]
    stop <- FALSE stop-if-true
    # "hopper wall=right 1"
    # "shifter=right 2"
    # "gear intake= xbox"
    # "left joystick\nconv+upt=0"
    # "ball intake=0 left"
    # "xboxY"
    # "gear shifts on bottom\nif not, button 2 on each side\nleft=low\nright=hi"
    # "Right Joystick:\nleft/right\nTrigger= intake motors fwd\nbottom= shift hi\n2= intake pistons or shift hi\n3= intake pistons?"
    # "Left Joystick:\nfwd/rev\nTrigger= conv+upt\nbottom= shift low\n2=shift low"
    # "xboxRB"
    # "xboxLB"
    # "xboxX"
    # "xboxB"
    # "xboxA"
    # "JOYSTICKS & CONTROLLER"
    # "RightJoystick"
    n143 = call <vilib>:"WPI_JoystickGetValues.vi"("JoystickDevRef"=w272) -> ("Buttons"=w273:bool[], "Axes"=w249:dbl[])  [unwired: 6 in, 3 out]
    n144 = Unbundle By Name(w288) -> ("JoystickDevRef"=w267:T10)
    n145 = call <vilib>:"WPI_JoystickGetValues.vi"("JoystickDevRef"=w285) -> ("Buttons"=w281:bool[], "Axes"=w284:dbl[])  [unwired: 6 in, 3 out]
    n146 = Array To Cluster(array=w273) -> (cluster=w274:T24)
    n147 = Array To Cluster(array=w284) -> (cluster=w283:T25)
    n148 = Array To Cluster(array=w281) -> (cluster=w282:T24)
    n149 = Array To Cluster(array=w249) -> (cluster=w248:T25)
    n150 = call <vilib>:"WPI_JoystickGetValues.vi"("JoystickDevRef"=w267) -> ("Buttons"=w268:bool[], "Axes"=w270:dbl[])  [unwired: 6 in, 3 out]
    n151 = Array To Cluster(array=w268) -> (cluster=w269:T24)
    n152 = Unbundle By Name(w248) -> ("Axes[2]"=w247:dbl, "Axes[3]"=w246:dbl)
    n153 = Array To Cluster(array=w270) -> (cluster=w271:T25)
    n154 = Unbundle By Name(w274) -> ("Buttons[0]"=w237:bool, "Buttons[1]"=w238:bool, "Buttons[2]"=w255:bool, "Buttons[4]"=w257:bool, "Buttons[5]"=w236:bool)  [unwired: 1 out]
    n155 = Unbundle By Name(w283) -> ("Axes[1]"=w276:dbl)
    n156 = Unbundle By Name(w269) -> ("Buttons[1]"=w233:bool, "Buttons[2]"=w241:bool)  [unwired: 5 out]
    n157 = Unbundle By Name(w282) -> ("Buttons[0]"=w252:bool, "Buttons[6]"=w250:bool)  [unwired: 4 out]
    n158 = Unbundle By Name(w271) -> ("Axes[0]"=w232:dbl)
    n159 = Negate(x=w276) -> (-x=w231:dbl)
    n160 = global read "Robot Global Data.vi" "Robot Mode"() -> (w243:T26)
    n161 = disable-structure shown="Disabled" {
      disable-tunnel: _ -> [w296 _]
      disable-tunnel: [w295 _] -> _
      frame Disabled {
        n162 = call "Joystick Stiction Compensation.vi"("A"="ANG-A", "B"="ANG-B", "Input"=w296) -> ("Output"=w295:dbl)  [unwired: 8 in]
        "ANG-Output" <- w295
        "ANG-Input" <- w296
      }
      frame Enabled {
      }
    }
    n163 = disable-structure shown="Disabled" {
      disable-tunnel: _ -> [w292 _]
      disable-tunnel: [w291 _] -> _
      frame Disabled {
        n164 = call "Joystick Stiction Compensation.vi"("A"="FWD-A", "B"="FWD-B", "Input"=w292) -> ("Output"=w291:dbl)  [unwired: 8 in]
        "FWD-Output" <- w291
        "FWD-Input" <- w292
      }
      frame Enabled {
      }
    }
    n165 = Equal?(x=w243, y=Control_1."Teleop Enabled") -> (x = y?=w253:bool)
    n166 = Not Equal?(x=w243, y=Control_1."Autonomous Enabled") -> (x != y?=w286:bool)
    n167 = case shown="True" w286 {
      tunnel: [w323 w357] -> w277
      tunnel: [w324 w360] -> w287
      tunnel: [w322 w355] -> w278
      tunnel: w232 -> [_ w356]
      tunnel: [w321 w359] -> w279
      tunnel: [w320 w354] -> w266
      tunnel: [w319 w352] -> w265
      tunnel: [w318 w350] -> w264
      tunnel: [w317 w349] -> w263
      tunnel: [w316 w347] -> w262
      tunnel: [w315 w346] -> w261
      tunnel: w255 -> [_ w353]
      tunnel: w252 -> [_ w351]
      tunnel: [FALSE w345] -> w260
      tunnel: w233 -> [_ w348]
      tunnel: [FALSE ("Output") w344] -> w259
      tunnel: w231 -> [_ w358]
      tunnel: [FALSE w342] -> w258
      tunnel: [FALSE w341] -> w235
      tunnel: w257 -> [_ w343]
      tunnel: w257 -> [_ _]
      tunnel: w237 -> [_ w340]
      tunnel: [w312 w339] -> w256
      tunnel: w253 -> [_ w331]
      tunnel: w241 -> [_ w338]
      tunnel: [TRUE w337] -> w251
      tunnel: w250 -> [_ w336]
      tunnel: w247 -> [_ w335]
      tunnel: w246 -> [_ w332]
      tunnel: [0.0 ("AutoDistance") w333] -> w245
      tunnel: [0.0 ("AutoDistance") w334] -> w244
      tunnel: [w306 w330] -> w242
      tunnel: [w305 w329] -> w240
      tunnel: [FALSE w328] -> w239
      tunnel: w238 -> [_ w327]
      tunnel: w236 -> [_ w326]
      tunnel: [FALSE ("GearIntakeCmd") w325] -> w234
      frame False {
        # "Autonomous Enabled"
        n168 = global read "Robot Global Data.vi" "AutoHopperPanelPistons"() -> (w317:bool)
        n169 = global read "Robot Global Data.vi" "AutoIntakePistons"() -> (w316:bool)
        n170 = global read "Robot Global Data.vi" "AutoFlyw"() -> (w320:bool)
        n171 = global read "Robot Global Data.vi" "AutoXAxis"() -> (w322:dbl)
        n172 = global read "Robot Global Data.vi" "AutoYAxis"() -> (w323:dbl)
        n173 = global read "Robot Global Data.vi" "AutoAngle"() -> (w324:dbl)
        n174 = global read "Robot Global Data.vi" "AutoDistance"() -> (w321:dbl)
        n175 = global read "Robot Global Data.vi" "AutoConv+Upt"() -> (w319:bool)
        n176 = global read "Robot Global Data.vi" "AutoIntakeRev"() -> (w315:bool)
        n177 = global read "Robot Global Data.vi" "AutoGearClamp"() -> (w318:bool)
        n178 = global read "Robot Global Data.vi" "AutoBallIntake"() -> (w306:bool)
        n179 = global read "Robot Global Data.vi" "AutoGyroReset"() -> (w305:bool)
        n180 = global read "Robot Global Data.vi" "AutoAngle PIDOn"() -> (w312:bool)
      }
      frame True {
        # "Not Autonomous"
        n181 = case shown="True" w331 {
          tunnel: [0.0 ("Axes[0]") "DriveAngleCmd"] -> w360
          tunnel: [0.0 ("Axes[0]") "DriveDistance Cmd"] -> w359
          tunnel: [0.0 ("Axes[0]") w409] -> w357
          tunnel: w358 -> [_ w409]
          tunnel: w356 -> [_ w408]
          tunnel: [0.0 ("Axes[0]") w408] -> w355
          tunnel: [FALSE ("Output") w392] -> w354
          tunnel: w353 -> [_ w393]
          tunnel: [FALSE ("Output") w406] -> w352
          tunnel: w351 -> [_ w405]
          tunnel: [TRUE ("Output") w390] -> w350
          tunnel: w348 -> [_ w385]
          tunnel: [TRUE ("Output") w383] -> w349
          tunnel: [FALSE ("Output") w384] -> w347
          tunnel: [FALSE ("Output") "CtrlIntakeReverse"] -> w346
          tunnel: [FALSE ("Output") "CtrlConv+UptReverse"] -> w345
          tunnel: [FALSE ("Output") w403] -> w344
          tunnel: w343 -> [_ w407]
          tunnel: [FALSE ("Output") w407] -> w342
          tunnel: [FALSE ("Output") w386] -> w341
          tunnel: w340 -> [_ w386]
          tunnel: [FALSE ("Output") FALSE] -> w339
          tunnel: w338 -> [_ w404]
          tunnel: [FALSE w402] -> w337
          tunnel: w336 -> [_ w401]
          tunnel: [0.0 ("Axes[2]") w399] -> w334
          tunnel: w335 -> [_ w399]
          tunnel: [0.0 ("Axes[5]") w398] -> w333
          tunnel: w332 -> [_ w398]
          tunnel: [FALSE ("Output") w395] -> w330
          tunnel: w326 -> [_ w394]
          tunnel: [FALSE ("Output") w387] -> w328
          tunnel: [FALSE ("Output") FALSE ("Output")] -> w329
          tunnel: w327 -> [_ w387]
          tunnel: [FALSE ("GearIntakeCmd") w388] -> w325
          frame False {
            # "Teleop Disabled"
          }
          frame True {
            # "GearIntakeCmd"
            # "Teleop Enabled"
            n182 = global read "Robot Global Data.vi" "GearPickupPistonsCmd"() -> (w384:bool)
            n183 = global read "Robot Global Data.vi" "GearClampCmd"() -> (w390:bool)
            n184 = global read "Robot Global Data.vi" "CtrlGearIntake"() -> (w388:bool)
            n185 = call "Toggle.vi"("Input"=w394) -> ("Output"=w395:bool)
            n186 = call "Toggle.vi"("Input"=w393) -> ("Output"=w392:bool)
            n187 = call "Toggle.vi"("Input"=w405) -> ("Output"=w406:bool)
            n188 = call "Toggle.vi"("Input"=w404) -> ("Output"=w403:bool)
            n189 = call "Toggle.vi"("Input"=w401) -> ("Output"=w402:bool)
            n190 = call "Toggle.vi"("Input"=w385) -> ("Output"=w389:bool)
            n191 = Not(x=w389) -> (.not. x?=w383:bool)
          }
        }
      }
    }
    n192 = global write "Robot Global Data.vi" "CtrlFlyw"(w266) -> ()
    n193 = global write "Robot Global Data.vi" "CtrlShiftHi"(w259) -> ()
    n194 = global write "Robot Global Data.vi" "DriveYaxis"(w277) -> ()
    n195 = global write "Robot Global Data.vi" "CtrlShiftLow"(w251) -> ()
    n196 = global write "Robot Global Data.vi" "GyroReset"(w240) -> ()
    n197 = global write "Robot Global Data.vi" "DriveXaxis"(w278) -> ()
    n198 = global write "Robot Global Data.vi" "DriveAngle"(w287) -> ()
    n199 = global write "Robot Global Data.vi" "CtrlConv+Upt"(w265) -> ()
    n200 = global write "Robot Global Data.vi" "AnglePIDOn"(w256) -> ()
    n201 = global write "Robot Global Data.vi" "CtrlBallIntake"(w242) -> ()
    n202 = global write "Robot Global Data.vi" "CtrlIntakeRev"(w261) -> ()
    n203 = global write "Robot Global Data.vi" "DriveDistance"(w279) -> ()
    n204 = global write "Robot Global Data.vi" "CtrlGearClamp"(w264) -> ()
    n205 = global write "Robot Global Data.vi" "CtrlConv+UptRev"(w260) -> ()
    n206 = global write "Robot Global Data.vi" "CtrlClimberMotor"(w258) -> ()
    n207 = global write "Robot Global Data.vi" "XBoxLeftTrigger"(w244) -> ()
    n208 = global write "Robot Global Data.vi" "CtrlGearPickupPistons"(w262) -> ()
    n209 = global write "Robot Global Data.vi" "XBoxRightTrigger"(w245) -> ()
    n210 = global write "Robot Global Data.vi" "CtrlHopperPanelPistons"(w263) -> ()
    n211 = global write "Robot Global Data.vi" "GearPickup"(w239) -> ()
    n212 = global write "Robot Global Data.vi" "CtrlGearIntake"(w234) -> ()
    n213 = global write "Robot Global Data.vi" "GearDrop"(w235) -> ()
    n214 = disable-structure shown="Disabled" {
      frame Disabled {
        n215 = feedback #1() -> (w300)  [unwired: 1 in]
        n216 = feedback-in #1() -> (w301)
        n217 = Not(x=w300) -> (.not. x?=w299:bool)
        n218 = And(y=w299) -> (x=w302:bool)  [unwired: 1 out]
      }
      frame Enabled {
      }
    }
    n219 = call "Elapsed Times.vi"("Call Name"="Joystick  Loop") -> ()  [unwired: 2 in, 1 out]
    n220 = Wait (ms)(milliseconds to wait=u32 100) -> ()  [unwired: 1 out]
  }
  n221 = while {
    tunnel: w11 -> [w442]
    tunnel: w9 -> [w421]
    tunnel: w8 -> [w417]
    stop <- FALSE stop-if-true
    # "SENSORS"
    # "4.16667 for 500 cnt /rev encoders - practice bot"
    # "1 for 120 cnt /rev encoders - competition bot"
    # "SENSORS"
    n222 = global read "Robot Global Data.vi" "DTResetEncoder"() -> (w426:bool)
    n223 = call <vilib>:"WPI_CANTalonSRX_ConfigStatusFrameRate.vi"("CAN Talon SRX Ref"=w421, "Talon SRX Status Frame"=WPI_CANTalonSRX_StatusFrame."General Status Frame", "Frame Rate Ms"=u32 10) -> ("CAN Talon SRX Ref"=w424:T6)  [unwired: 12 in]
    n224 = Or(x=w426, y="DT Encoder Reset") -> (x .or. y?=w422:bool)
    n225 = call <vilib>:"WPI_CANTalonSRX_ConfigStatusFrameRate.vi"("CAN Talon SRX Ref"=w417, "Talon SRX Status Frame"=WPI_CANTalonSRX_StatusFrame."General Status Frame", "Frame Rate Ms"=u32 10) -> ("CAN Talon SRX Ref"=w416:T6)  [unwired: 12 in]
    n226 = global read "Robot Global Data.vi" "GyroReset"() -> (w444:bool)
    n227 = case shown="True" w422 {
      tunnel: w424 -> [w453 w458]
      tunnel: [w453 w457] -> w423
      tunnel: w416 -> [w452 w455]
      tunnel: [w452 w454] -> w415
      frame False {
      }
      frame True {
        n228 = call <vilib>:"WPI_CANTalonSRX_SetSensorPosition.vi"("New Sensor Position"=0.0, "CAN Talon SRX Ref"=w458) -> ("CAN Talon SRX Ref"=w457:T6)  [unwired: 8 in, 1 out]
        n229 = call <vilib>:"WPI_CANTalonSRX_SetSensorPosition.vi"("New Sensor Position"=0.0, "CAN Talon SRX Ref"=w455) -> ("CAN Talon SRX Ref"=w454:T6)  [unwired: 8 in, 1 out]
      }
    }
    n230 = Or(x=w444, y="Reset Gyro") -> (x .or. y?=w445:bool)
    n231 = call <vilib>:"WPI_CANTalonSRX_GetStatus.vi"("CAN Talon SRX Ref"=w423) -> ("Talon SRX Status"=w429:T20)  [unwired: 8 in, 2 out]
    n232 = case shown="True" w445 {
      tunnel: [w460 w462] -> w447
      tunnel: w442 -> [w460 w461]
      frame False {
      }
      frame True {
        n233 = call <vilib>:"WPI_GyroReset.vi"("GyroDevRef"=w461) -> ("GyroDevRef"=w462:T16)  [unwired: 9 in, 1 out]
      }
    }
    n234 = call <vilib>:"WPI_CANTalonSRX_GetStatus.vi"("CAN Talon SRX Ref"=w415) -> ("Talon SRX Status"=w440:T20)  [unwired: 8 in, 2 out]
    n235 = Unbundle By Name(w429) -> ("Sensor Position"=w420:dbl)
    n236 = Unbundle By Name(w440) -> ("Sensor Position"=w413:dbl)
    n237 = call <vilib>:"WPI_GyroGetAngle.vi"("GyroDevRef"=w447) -> ("Angle"=w441:dbl)  [unwired: 6 in, 4 out]
    "Gyro Angle" <- w441
    n238 = Divide(x=w413, y=1.0) -> (x/y=w412:dbl)
    "DT Right Distance" <- w412
    n239 = Divide(x=w420, y=1.0) -> (x/y=w430:dbl)
    "DT Left Distance" <- w430
    n240 = Add(x=w430, y=w412) -> (x+y=w439:dbl)
    n241 = global write "Robot Global Data.vi" "GyroYaw(Deg)"(w441) -> ()
    n242 = global write "Robot Global Data.vi" "DTLeftEncPos"(w430) -> ()
    n243 = Divide(x=w439, y=2.0) -> (x/y=w435:dbl)
    "DT Encoder Avg" <- w435
    n244 = global read "Robot Global Data.vi" "DriveDistance"() -> (w436:dbl)
    n245 = global write "Robot Global Data.vi" "DTRightEncPos"(w412) -> ()
    n246 = global read "Robot Global Data.vi" "DriveAngle"() -> (w446:dbl)
    n247 = global write "Robot Global Data.vi" "DTEncoder Avg"(w435) -> ()
    n248 = Bundle("DriveAngle"=w446, "Angle"=w441) -> (→"Yaw Cmd & Angle":cluster{"DriveAngle":dbl, "Angle":dbl})  [unwired: 1 in]
    n249 = Subtract(x=w430, y=w412) -> (x-y=→"DT Encoder L-R":dbl)
    n250 = Bundle("DriveDistance"=w436, w435) -> (→"DT Forward Cmd & Avg Distance":cluster{"DriveDistance":dbl, dbl})  [unwired: 1 in]
    n251 = Bundle("DriveDistance"=w436, w412) -> (→"DT Fwd Cmd & Right Encoder":cluster{"DriveDistance":dbl, dbl})  [unwired: 1 in]
    n252 = Bundle("DriveDistance"=w436, w430) -> (→"DT Fwd Cmd & Left Encoder":cluster{"DriveDistance":dbl, dbl})  [unwired: 1 in]
    n253 = call "Elapsed Times.vi"("Call Name"="Sensor Loop") -> ()  [unwired: 2 in, 1 out]
    n254 = Wait (ms)(milliseconds to wait=u32 20) -> ()  [unwired: 1 out]
  }
